vi "EV Rotator Control Disengage Motors Editor.vi"(6 "Channel":i32=1, 8 "Calibration in":string, 9 "Hardware in":string, 10 "Setup in":string, 11 "Editor seq info":T1 {"Steps config"."Loop Info"."unit scale" items=["Log", "Lin"]; "Steps config"."Loop Info"."unit dB ref" format="%#_6p"}) -> (1 "Step name out":string="Calibration Default", 2 "Setup out":string, 3 "Sequence channels & curves out":string[](array[string]))   [LabVIEW 2018]
uses:
  custom and Sc run Seq Sub VIs (x64).llb/Axis Unit Type.ctl
  G:/AP_Testing/Emma Dufresne/rotator/Custom VIs/EV.Rotator.RotatorControl.dll
  custom and Sc run Seq Sub VIs (x64).llb/editor seq info.ctl
  custom and Sc run Seq Sub VIs (x64).llb/Steps config.ctl
panel:
  out "RotatorControl.dll version":string
  in  "Function to run":enum16{"MoveDegrees", "EaseToEVCoords"}(ring)
  in  "Absolute mode":bool
  in  "Vertical/Meridians angle":dbl format="%.2f"
  in  "Horizontal/Parallels angle":dbl format="%.2f"
  in  "Save as":bool
  in  "save":bool
  in  "revert":bool
  in  "continue loop?":bool
  in  "cancel":bool
  in  "load":bool
  # "Note, VI looks for memory list values:\n - Horizontal Offset\n - Vertical Offset\n - Depth Offset\nto set rotation axis offsets (inches).\n\nIt also looks for memory list value:\n - VertCorrection\nas a fudge factor added to the calculated vertical axis angle sent to the rotator."
  # "Reminder:  You must edit this custom step from\nwithin a sequence for it to remember your settings."
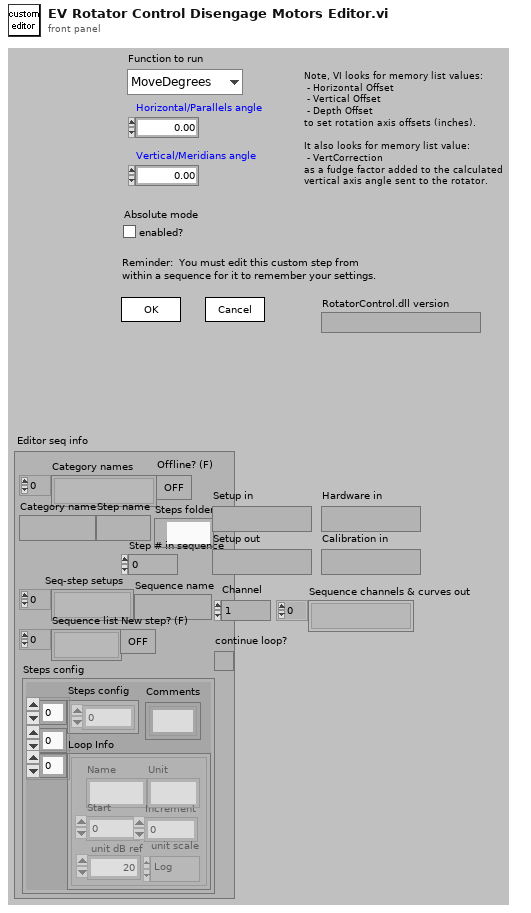
[diagram p1: front panel]
types:
  T1 = typedef "editor seq info.ctl" = cluster{"Category names":string[], "Category name":string, "Step name":string, "Step # in sequence":i32, "Seq-step setups":string[], "Sequence name":string, "Sequence list":string[], "New step? (F)":bool, "Steps config":T2, "Offline? (F)":bool, "Steps folder":path}
  T2 = typedef "Steps config.ctl" = cluster{"Steps config":i32[][], "Loop Info":cluster{"Name":string, "Start":dbl, "Increment":dbl, "Unit":string, "unit dB ref":dbl, "unit scale":u16}[], "Comments":string[]}
  T3 = cluster{"Horizontal/parallels angle":dbl, "Vertical/meridians angle":dbl, "Function to run":enum16{"MoveDegrees", "EaseToEVCoords"}, "Absolute position mode":bool}
  T4 = cluster{"load":bool, "revert":bool, bool, "cancel":bool, "Save as":bool, bool, bool}
  T5 = cluster{"load":bool, "revert":bool, "save":bool, "cancel":bool, "Save as":bool, "close panel":bool, "apply":bool}
  T6 = typedef "seq step setup.ctl" = cluster{"Input Signal Channels":i32[], "Output Signal Channels":i32[], "Curves selected":string[][], "Curves generated":string[], "Step setup flat":string, "Trigger Signal Channel":i32, "Curves Generated Assumptions":cluster{"seq-setup in":string, "Relevant subset of mem list Grouping":cluster{T7[]}[]}}
  T7 = typedef "Memory List Grouping.ctl" = cluster{"item name":string, "parent":string, "Open?":bool, "Type":T8}
  T8 = typedef "Memory List Grouping - Item Type.ctl" = enum16{"item", "custom group", "auto group", "protected group"}
  T9 = typedef "Axis Unit Type.ctl" = u16
  T10 = typedef "data cluster.ctl" = cluster{"Name":string, "Curve":cluster{"x":dbl, "y":dbl, "z":dbl}[], "X data":T9, "Y data":T9, "Z data":T9, "X axis":u16, "Y axis":u16, "Z axis":u16, "X unit":string, "Y unit":string, "Z unit":string, "X dB ref":dbl, "Y dB ref":dbl, "Z dB ref":dbl, "single val":bool, "protected":bool, "display X":bool, "display Y":bool, "display Z":bool, "Plot Settings":cluster{"Color":u32, "Interpolation":u8, "Point Style":u8, "Line Style":u8, "Point Color":u32, "Line Width":u8, "Bar Plot Style":u8, "Fill To":i16}, "Test Info":string}
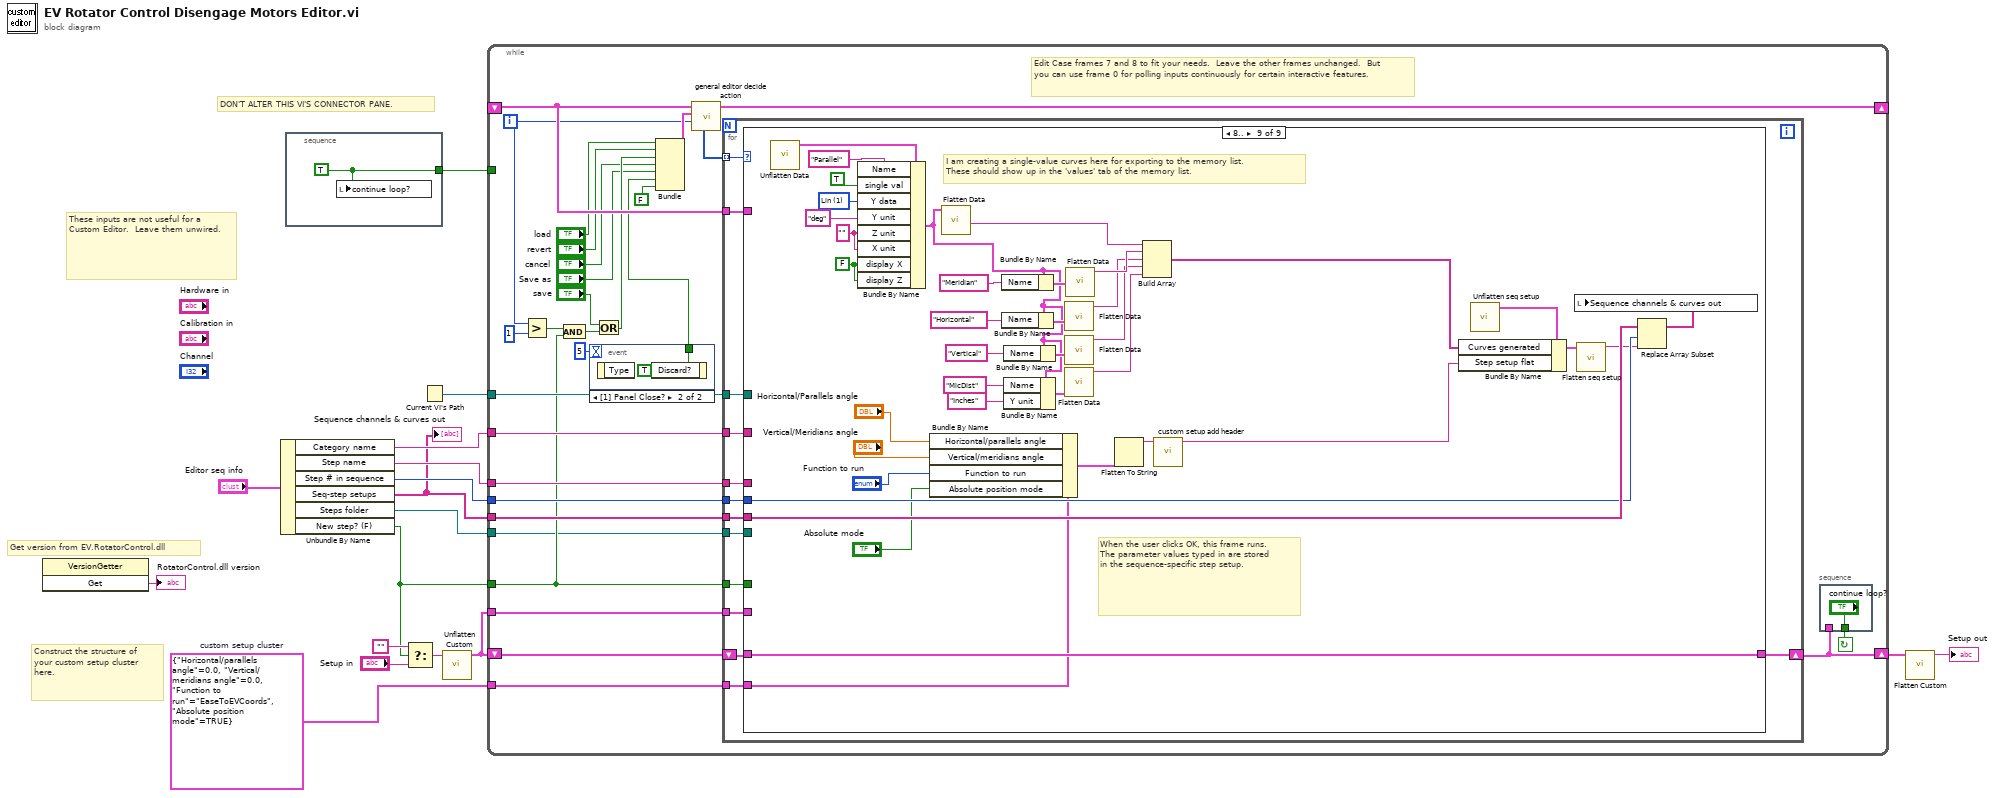
[diagram p0: block diagram]
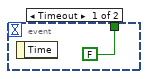
[diagram p2: hidden frame]
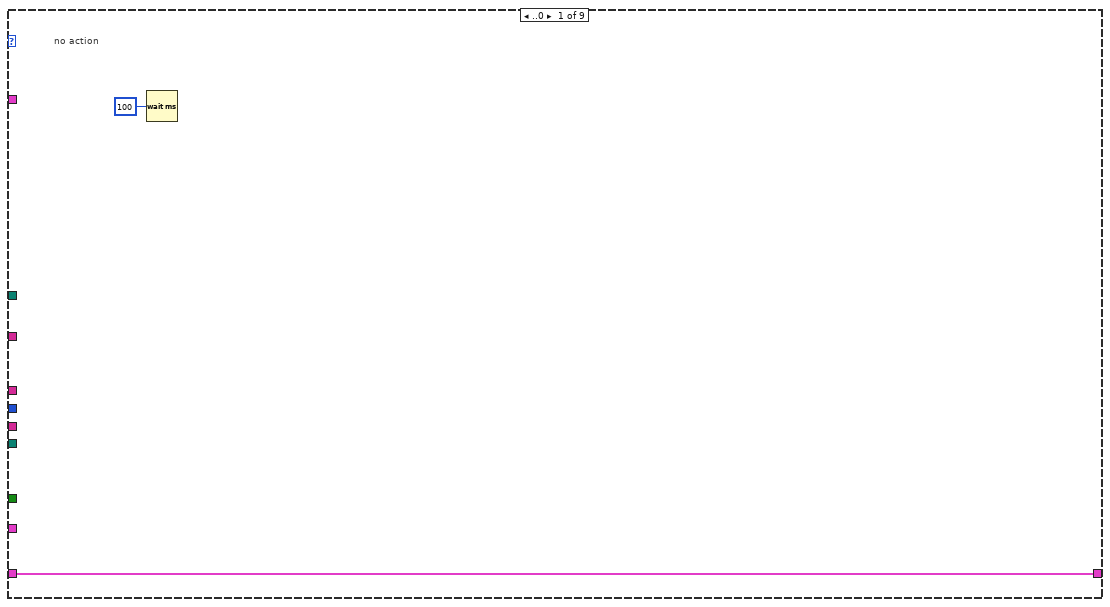
[diagram p3: hidden frame]
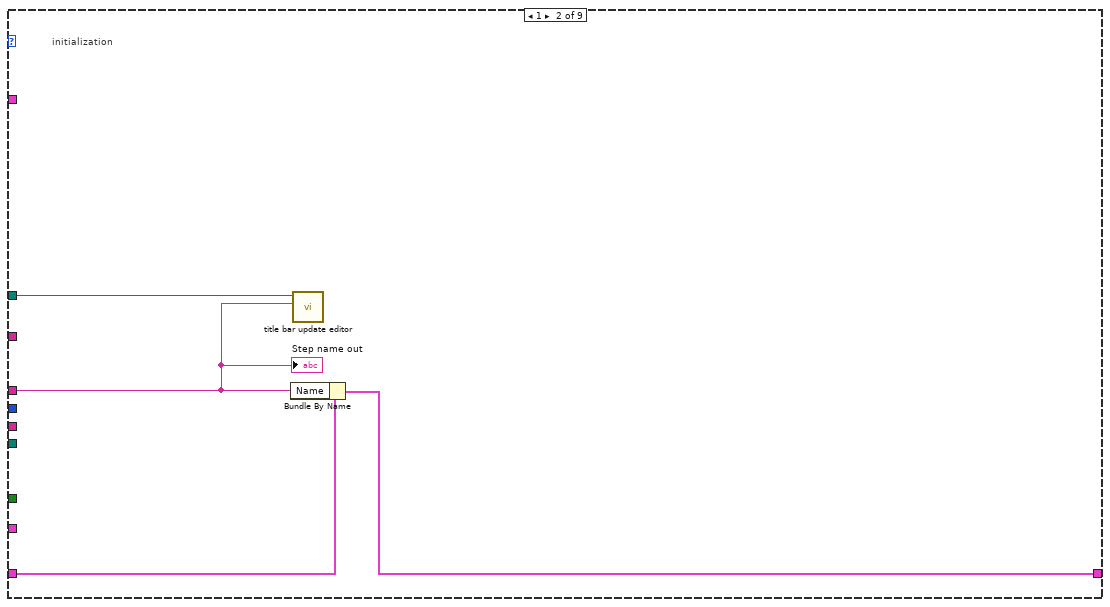
[diagram p4: hidden frame]
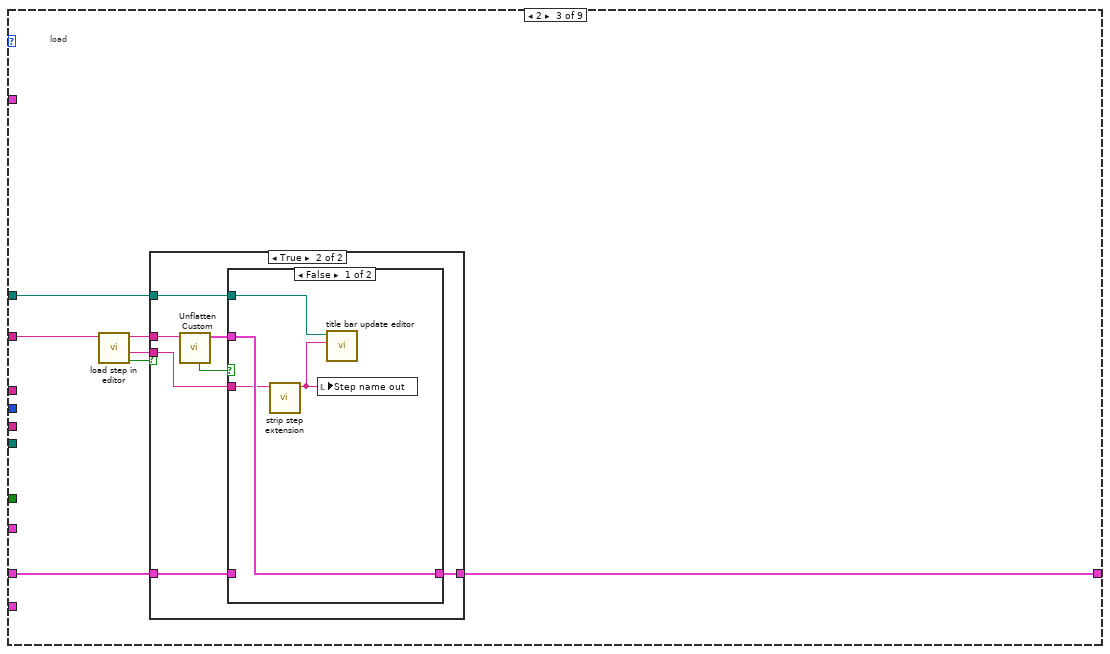
[diagram p5: hidden frame]
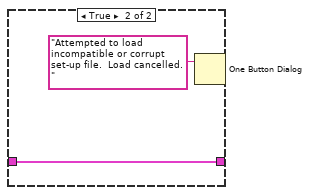
[diagram p7: hidden frame]
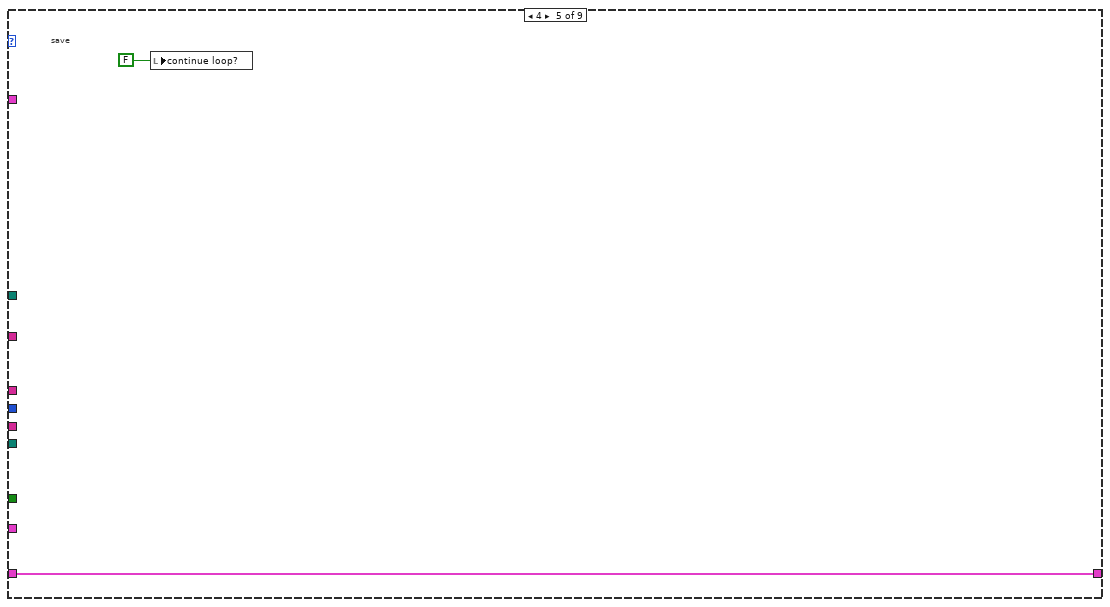
[diagram p9: hidden frame]
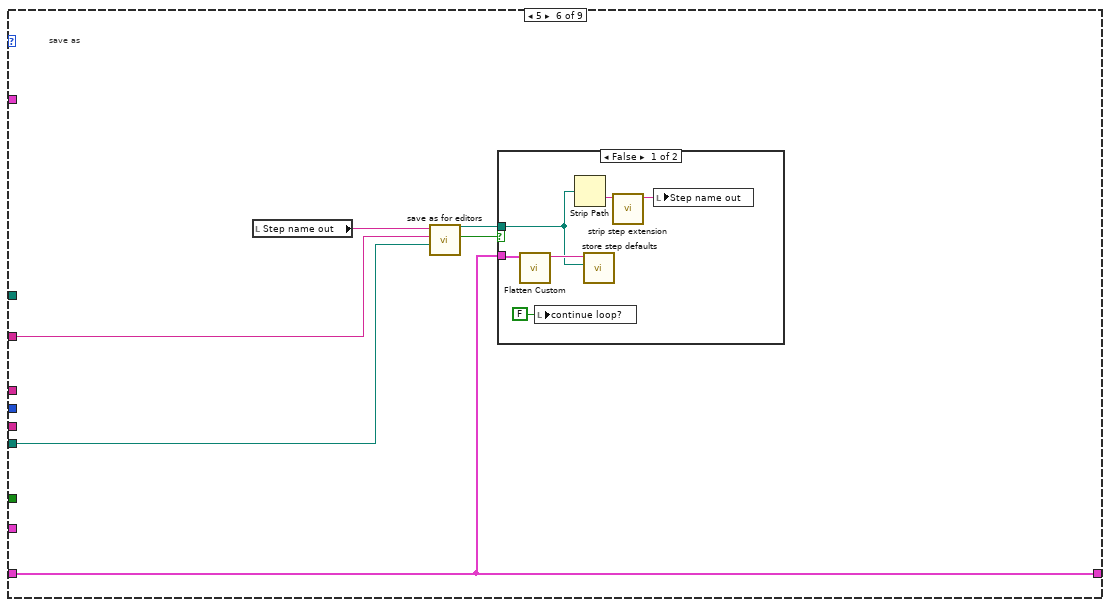
[diagram p10: hidden frame]
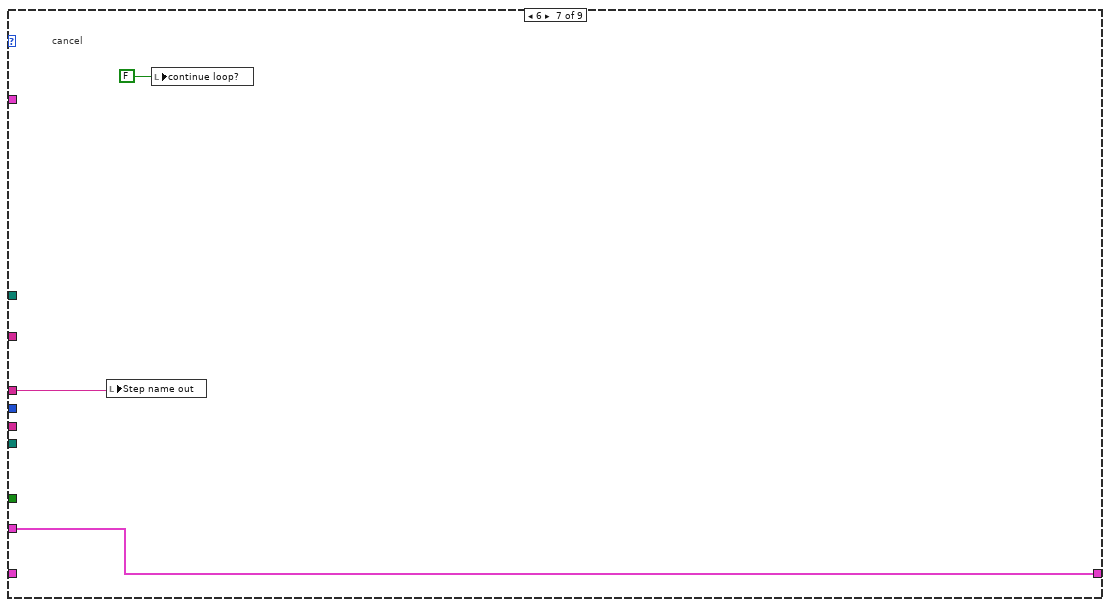
[diagram p12: hidden frame]
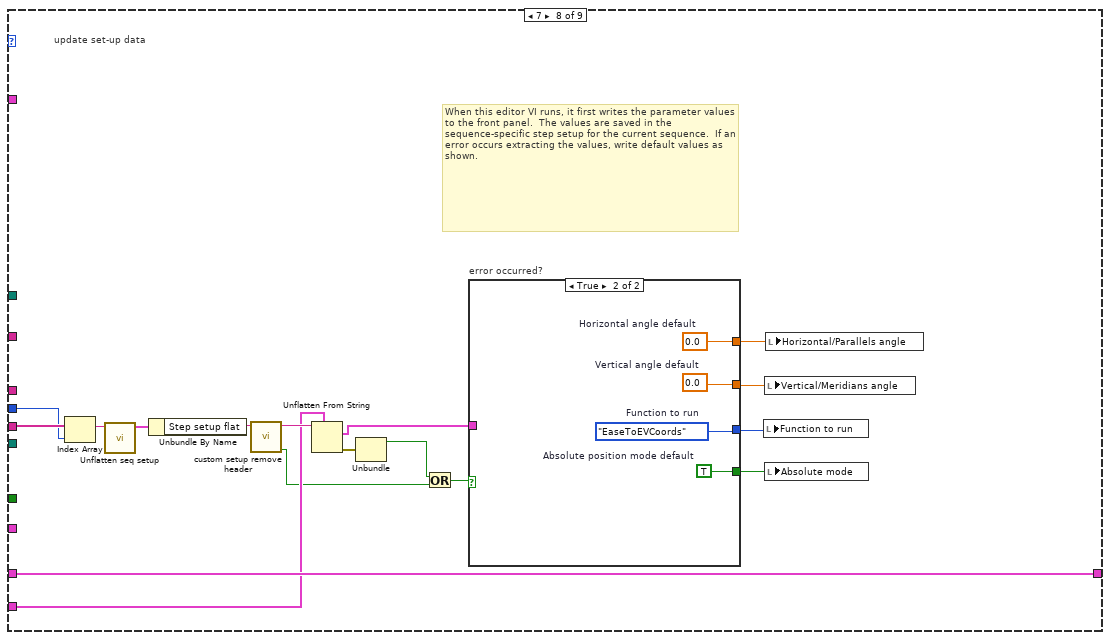
[diagram p13: hidden frame]
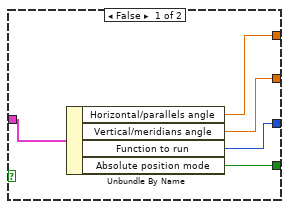
[diagram p14: hidden frame]
diagram:
  w13 = T3 {"Horizontal/parallels angle"=0.0, "Vertical/meridians angle"=0.0, "Function to run"=enum."EaseToEVCoords", "Absolute position mode"=TRUE}  # custom setup cluster
  # "Get version from EV.RotatorControl.dll"
  # "Construct the structure of your custom setup cluster here."
  # "These inputs are not useful for a Custom Editor.  Leave them unwired."
  # "DON'T ALTER THIS VI'S CONNECTOR PANE."
  n1 = invoke class="VersionGetter" method="Get"() -> ("Get"=→"RotatorControl.dll version":string)  [unwired: 3 in, 2 out]
  n2 = Unbundle By Name("Editor seq info") -> ("Category name"=w10:string, "Step name"=w9:string, "Step # in sequence"=w8:i32, "Seq-step setups"=w6:string[], "Steps folder"=w7:path, "New step? (F)"=w3:bool)
  "Sequence channels & curves out" <- w6
  n3 = stacked-sequence {
    tunnel: [w18] -> w11
    frame #0 {
      w18 = TRUE ("continue loop?")
      n4 = local write "continue loop?"(w18) -> ()
    }
  }
  n5 = Select(t="", s=w3, f="Setup in") -> (s? t:f=w14:string)
  n6 = Current VI's Path() -> (path=w12:path)
  n7 = call "Unflatten Custom.vi"("Unflatten Custom"=w14) -> ("Custom"=w2:cluster{"Name":string})  [unwired: 10 out]
  n8 = while {
    tunnel: w13 -> [w28]
    tunnel: w12 -> [w36]
    shift-left: w2 -> [w38]
    shift-right: [w29] -> w4
    tunnel: w2 -> [w40]
    tunnel: w3 -> [w32]
    tunnel: w6 -> [w42]
    tunnel: w8 -> [w43]
    tunnel: w9 -> [w44]
    tunnel: w10 -> [w45]
    shift-left: _ -> [w39]
    shift-right: [w47] -> _
    tunnel: w7 -> [w25]
    tunnel: w11 -> [_]
    i -> [w35]
    stop <- w41 continue-if-true
    # "Edit Case frames 7 and 8 to fit your needs.  Leave the other frames unchanged.  But you can use frame 0 for polling inputs continuously for certain interactive features."
    n9 = Greater?(x=w35, y=1) -> (0:w33:bool)
    n10 = And(x=w33, y=w32) -> (x .and. y?=w31:bool)
    n11 = event shown="[1] Panel Close?" {
      selector: _ -> [_ _]
      dyn-events: _ -> [_ _]
      timeout: 5 -> [_ _]
      tunnel: [FALSE w49] -> w27
      event Timeout {
        n12 = event-data() -> ()  [unwired: 2 out]
      }
      event Panel Close? {
        w49 = TRUE
        n13 = event-data() -> ()  [unwired: 2 out]
        n14 = event-data("Discard?"=w49) -> ()  [unwired: 1 in, 1 out]
      }
    }
    n15 = Or(x="save", y=w31) -> (x .or. y?=w30:bool)
    n16 = Bundle("load"="load", "revert"="revert", w30, "cancel"="cancel", "Save as"="Save as", w27, FALSE) -> (w37:T4)  [unwired: 1 out]
    n17 = call "general editor decide action.vi"("Iteration"=w35, "Polled cluster"=w37, "Old cluster"=w39) -> ("actions array"=w46:i32[], "New cluster"=w47:T5)  [unwired: 1 in, 6 out]
    n18 = for {
      tunnel: w39 -> [w63]
      tunnel: w40 -> [w62]
      tunnel: w32 -> [w61]
      tunnel: w42 -> [w60]
      tunnel: w43 -> [w59]
      tunnel: w44 -> [w58]
      tunnel: w45 -> [w57]
      tunnel: w46 -> [w56] mode=indexing
      shift-right: [w54] -> w29
      shift-left: w38 -> [w55]
      tunnel: w36 -> [w53]
      tunnel: w28 -> [w52]
      tunnel: w25 -> [w51]
      n19 = case shown="8.." w56 {
        tunnel: w57 -> [_ _ w72 _ _ w96 _ _ _]
        tunnel: w58 -> [_ w66 _ _ _ _ w106 _ _]
        tunnel: w59 -> [_ _ _ _ _ _ _ w122 w169]
        tunnel: w60 -> [_ _ _ _ _ _ _ w123 w170]
        tunnel: w61 -> [_ _ _ _ _ _ _ _ _]
        tunnel: w62 -> [_ _ _ w91 _ _ w107 _ _]
        tunnel: [w64 w69 w76 w91 w92 w99 w107 w125 w166] -> w54
        tunnel: w55 -> [w64 w68 w75 _ w92 w99 _ w125 w166]
        tunnel: w63 -> [_ _ _ _ _ _ _ _ _]
        tunnel: w53 -> [_ w67 w70 _ _ _ _ _ _]
        tunnel: w52 -> [_ _ _ _ _ _ _ w118 w163]
        tunnel: w51 -> [_ _ _ _ _ w94 _ _ _]
        frame ..0 {
          # "no action"
          n20 = Wait (ms)(milliseconds to wait=u32 100) -> ()  [unwired: 1 out]
        }
        frame 1 {
          # "initialization"
          n21 = Bundle By Name(cluster=w68, "Name"=w66) -> (w69:cluster{"Name":string})
          n22 = call "title bar update editor.vi"("Step name"=w66, "Editor VI path"=w67) -> ()  [unwired: 10 out]
          "Step name out" <- w66
        }
        frame 2 {
          # "load"
          n23 = call "load step in editor.vi"("Category name"=w72) -> ("Not canceled?"=w73:bool, "New step name (with ext.)"=w71:string, "Flat step set-up"=w74:string)  [unwired: 1 in, 7 out]
          n24 = case shown="True" w73 {
            tunnel: w74 -> [_ w84]
            tunnel: [w77 w82] -> w76
            tunnel: w75 -> [w77 w81]
            tunnel: w71 -> [_ w79]
            tunnel: w70 -> [_ w78]
            frame False {
            }
            frame True {
              n25 = call "Unflatten Custom.vi"("Unflatten Custom"=w84) -> ("Custom"=w80:cluster{"Name":string}, "Error?"=w83:bool)  [unwired: 9 out]
              n26 = case shown="False" w83 {
                tunnel: [w88 w90] -> w82
                tunnel: w81 -> [_ w90]
                tunnel: w80 -> [w88 _]
                tunnel: w79 -> [w87 _]
                tunnel: w78 -> [w86 _]
                frame False {
                  n27 = call "strip step extension.vi"("Step name w/ extension"=w87) -> ("Step name (base)"=w85:string)  [unwired: 1 in, 9 out]
                  n28 = local write "Step name out"(w85) -> ()
                  n29 = call "title bar update editor.vi"("Step name"=w85, "Editor VI path"=w86) -> ()  [unwired: 10 out]
                }
                frame True {
                  n30 = One Button Dialog(message="Attempted to load incompatible or corrupt set-up file.  Load cancelled.") -> ()  [unwired: 2 out]
                }
              }
            }
          }
        }
        frame 3 {
          # "revert"
        }
        frame 4 {
          # "save"
          n31 = local write "continue loop?"(FALSE ("continue loop?")) -> ()
        }
        frame 5 {
          # "save as"
          n32 = local read "Step name out"() -> (w95:string)
          n33 = call "save as for editors.vi"("Steps Folder (gbl if empty)"=w94, "Category name"=w96, "Step name"=w95) -> ("Canceled"=w97:bool, "File path chosen"=w98:path)  [unwired: 3 in, 4 out]
          n34 = case shown="False" w97 {
            tunnel: w98 -> [w101 _]
            tunnel: w99 -> [w104 _]
            frame False {
              n35 = call "Flatten Custom.vi"("Custom"=w104) -> ("Custom flattened"=w105:string)  [unwired: 10 out]
              n36 = local write "continue loop?"(FALSE ("continue loop?")) -> ()
              n37 = Strip Path(path=w101) -> (name=w102:string)  [unwired: 1 out]
              n38 = call "store step defaults.vi"("Set-up file"=w101, "Flat step set-up"=w105) -> ()  [unwired: 4 in, 6 out]
              n39 = call "strip step extension.vi"("Step name w/ extension"=w102) -> ("Step name (base)"=w100:string)  [unwired: 1 in, 9 out]
              n40 = local write "Step name out"(w100) -> ()
            }
            frame True {
            }
          }
        }
        frame 6 {
          # "cancel"
          n41 = local write "Step name out"(w106) -> ()
          n42 = local write "continue loop?"(FALSE ("continue loop?")) -> ()
        }
        frame 7 {
          # "When this editor VI runs, it first writes the parameter values to the front panel.  The values are saved in the sequence-specific step setup for the current sequence.  If an error occurs extracting the values, write default values as shown."
          # "update set-up data"
          n43 = Index Array(array=w123, index=w122) -> (element=w124:string)
          n44 = call "Unflatten seq setup.vi"("Unflatten seq setup"=w124) -> ("Sequence-specific step set-up"=w121:T6)  [unwired: 3 in, 7 out]
          n45 = Unbundle By Name(w121) -> ("Step setup flat"=w120:string)
          n46 = call "custom setup remove header.vi"("Output from 'Step setup flat' of seq-setup structure"=w120) -> ("Error?"=w117:bool, "Flattened custom step setup cluster"=w119:string)  [unwired: 9 out]
          n47 = Unflatten From String(type=w118, binary string=w119) -> (value=w114:T3, error out=w111:errorcluster)  [unwired: 1 in, 3 out]
          n48 = Unbundle(w111) -> ("status"=w116:bool)  [unwired: 2 out]
          n49 = Or(x=w116, y=w117) -> (x .or. y?=w115:bool)
          n50 = case "error occurred?" shown="True" w115 {
            tunnel: w114 -> [w130 _]
            tunnel: [w129 w133] -> w113
            tunnel: [w128 w134] -> w112
            tunnel: [w127 w131] -> w110
            tunnel: [w126 w132] -> w109
            frame False {
              n51 = Unbundle By Name(w130) -> ("Horizontal/parallels angle"=w128:dbl, "Vertical/meridians angle"=w129:dbl, "Function to run"=w127:enum16{"MoveDegrees", "EaseToEVCoords"}, "Absolute position mode"=w126:bool)
            }
            frame True {
              w131 = enum16{"MoveDegrees", "EaseToEVCoords"}."EaseToEVCoords"  # Function to run
              w132 = TRUE  # Absolute position mode default
              w133 = 0.0  # Vertical angle default
              w134 = 0.0  # Horizontal angle default
            }
          }
          n52 = local write "Function to run"(w110) -> ()
          n53 = local write "Vertical/Meridians angle"(w113) -> ()
          n54 = local write "Absolute mode"(w109) -> ()
          n55 = local write "Horizontal/Parallels angle"(w112) -> ()
        }
        frame 8.. {
          w136 = T9 1 items=["dB", "Lin", "Pwr"] ("Y data")
          w137 = FALSE ("display X")
          w138 = "" ("Z unit")
          # "I am creating a single-value curves here for exporting to the memory list.\nThese should show up in the 'values' tab of the memory list."
          # "When the user clicks OK, this frame runs.  The parameter values typed in are stored in the sequence-specific step setup."
          n56 = call "Unflatten Data.vi"() -> ("Datum"=w156:T10)  [unwired: 1 in, 10 out]
          n57 = Bundle By Name(cluster=w156, "Name"="Parallel", "single val"=TRUE, "Y data"=w136, "Y unit"="deg" ("angle in degrees"), "Z unit"=w138, "X unit"=w138, "display X"=w137, "display Z"=w137) -> (w140:T10)
          n58 = Bundle By Name(cluster=w163, "Horizontal/parallels angle"="Horizontal/Parallels angle", "Vertical/meridians angle"="Vertical/Meridians angle", "Function to run"="Function to run", "Absolute position mode"="Absolute mode") -> (w162:T3)
          n59 = call "Flatten Data.vi"("Datum"=w140) -> ("Data flattened"=w158:string)  [unwired: 10 out]
          n60 = Bundle By Name(cluster=w140, "Name"="Meridian") -> (w152:T10)
          n61 = Bundle By Name(cluster=w140, "Name"="Horizontal") -> (w148:T10)
          n62 = Bundle By Name(cluster=w140, "Name"="Vertical") -> (w145:T10)
          n63 = Bundle By Name(cluster=w140, "Name"="MicDist", "Y unit"="Inches" ("X unit")) -> (w142:T10)
          n64 = call "Flatten Data.vi"("Datum"=w148) -> ("Data flattened"=w147:string)  [unwired: 10 out]
          n65 = call "Flatten Data.vi"("Datum"=w145) -> ("Data flattened"=w144:string)  [unwired: 10 out]
          n66 = call "Flatten Data.vi"("Datum"=w142) -> ("Data flattened"=w141:string)  [unwired: 10 out]
          n67 = call "Flatten Data.vi"("Datum"=w152) -> ("Data flattened"=w151:string)  [unwired: 10 out]
          n68 = Flatten To String(anything=w162) -> (data string=w164:string)  [unwired: 1 in, 4 out]
          n69 = Build Array(w158, w151, w147, w144, w141) -> (w159:string[])
          n70 = call "custom setup add header.vi"("Flattened custom step setup cluster"=w164) -> ("Input to 'Step setup flat' of seq-setup structure"=w165:string)  [unwired: 1 in, 9 out]
          n71 = call "Unflatten seq setup.vi"() -> ("Sequence-specific step set-up"=w172:T6)  [unwired: 4 in, 7 out]
          n72 = Bundle By Name(cluster=w172, "Curves generated"=w159, "Step setup flat"=w165) -> (w171:T6)
          n73 = call "Flatten seq setup.vi"("Sequence-specific step set-up"=w171) -> ("Seq setup flattened"=w168:string)  [unwired: 10 out]
          n74 = Replace Array Subset(array=w170, new element=w168, index=w169) -> (w167:string[])
          n75 = local write "Sequence channels & curves out"(w167) -> ()
        }
      }
    }
    n76 = stacked-sequence {
      tunnel: ["continue loop?"] -> w41
      tunnel: w29 -> [_]
      frame #0 {
      }
    }
  }
  n77 = call "Flatten Custom.vi"("Custom"=w4) -> ("Custom flattened"=→"Setup out":string)  [unwired: 10 out]
